vi "main_median_filter_update.vi"(8 "error in (no error)":errorcluster, 9 "Median Filtered Image":T1, 10 "Spaced Out Images":T1[](array[typedef]), 11 "Session In":T2) -> (0 "error out":errorcluster)   [LabVIEW 2019]
uses:
  <vilib>/userDefined/High Color/IMAQdx.ctl
  <vilib>/vision/Image Controls.llb/IMAQ Image.ctl
  <vilib>/vision/driver/IMAQdx.llb/IMAQdx Buffer Number Mode.ctl
  ParametersGlobal.vi
  DebugGlobal.vi
  <vilib>/vision/driver/NI_Vision_Acquisition_Software.lvlib
  <vilib>/vision/NI_Vision_Development_Module.lvlib
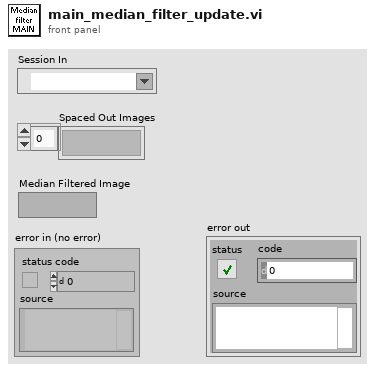
[diagram p1: front panel]
types:
  T1 = typedef "IMAQ Image.ctl" = refnum<image>
  T2 = typedef "IMAQdx.ctl" = refnum<k21>
  T3 = typedef "Image Type" = u32
  T4 = typedef "NI_Vision_Acquisition_Software.lvlib/IMAQdx Buffer Number Mode.ctl" = enum32{"Next", "Last", "Buffer Number", "Every", "Last New"}
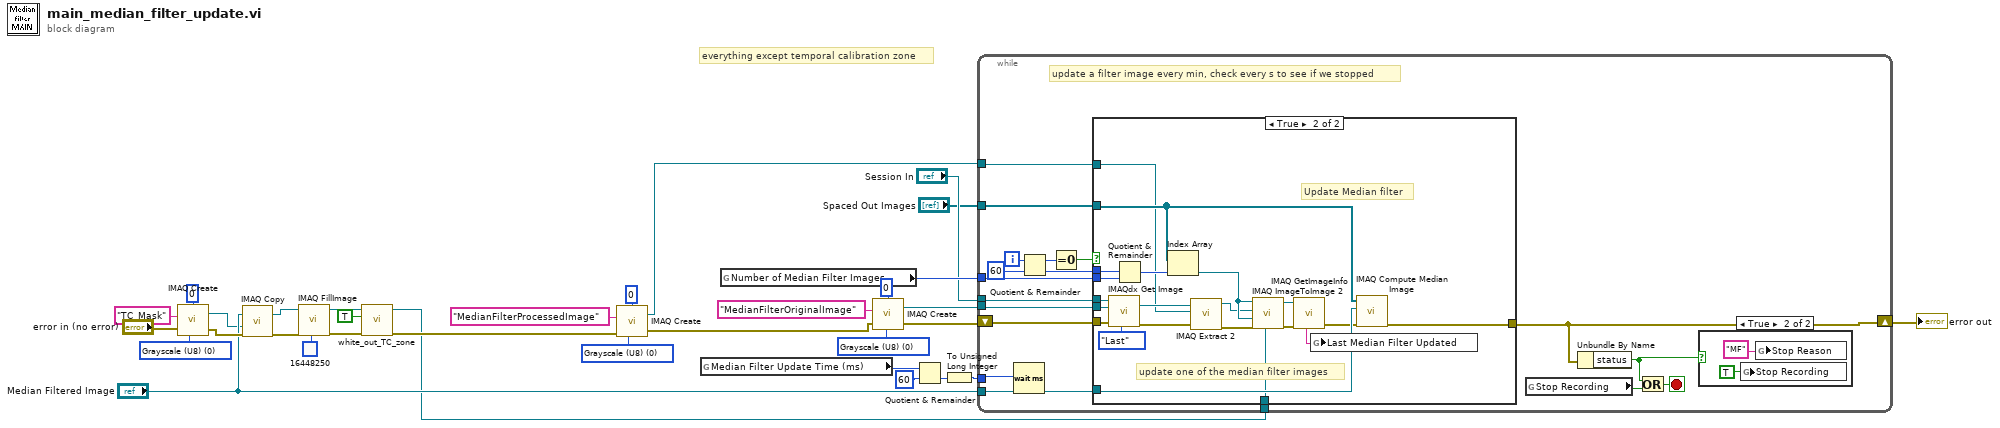
[diagram p0: block diagram]
diagram:
  w13 = T3 0 items=["Grayscale (U8)", "Grayscale (I16)", "Grayscale (SGL)", "Complex (CSG)", "RGB (U32)", "HSL (U32)", "RGB (U64)"] ("Image Type")
  w18 = T3 0 items=["Grayscale (U8)", "Grayscale (I16)", "Grayscale (SGL)", "Complex (CSG)", "RGB (U32)", "HSL (U32)", "RGB (U64)"] ("Image Type")
  w26 = T3 0 items=["Grayscale (U8)", "Grayscale (I16)", "Grayscale (SGL)", "Complex (CSG)", "RGB (U32)", "HSL (U32)", "RGB (U64)"] ("Image Type")
  # "everything except temporal calibration zone"
  n1 = call "IMAQ Create"("Border Size"=0, "Image Name"="TC_Mask", "Image Type"=w13, "error in (no error)"="error in (no error)") -> ("New Image"=w9:T1, "error out"=w11:errorcluster)  [unwired: 1 in]
  n2 = call "IMAQ Copy"("error in (no error)"=w11, "Image Dst"=w9, "Image Src"="Median Filtered Image") -> ("error out"=w7:errorcluster, "Image Dst Out"=w6:T1)  [unwired: 3 in]
  n3 = call "IMAQ FillImage"("Color Pixel Value"=u32 16448250, "error in (no error)"=w7, "Image"=w6) -> ("error out"=w4:errorcluster, "Image Out"=w3:T1)  [unwired: 7 in]
  n4 = call "white_out_TC_zone.vi"("error in (no error)"=w4, "Blackout?"=TRUE, "Refnum in"=w3) -> ("error out"=w2:errorcluster, "Refnum out"=w1:T1)  [unwired: 7 in]
  n5 = call "IMAQ Create"("Border Size"=0, "Image Name"="MedianFilterProcessedImage", "Image Type"=w18, "error in (no error)"=w2) -> ("New Image"=w16:T1, "error out"=w17:errorcluster)  [unwired: 1 in]
  n6 = global read "ParametersGlobal.vi" "Median Filter Update Time (ms)"() -> (w30:i32)
  n7 = global read "ParametersGlobal.vi" "Number of Median Filter Images"() -> (w29:i32)
  n8 = call "IMAQ Create"("Border Size"=0, "Image Name"="MedianFilterOriginalImage", "Image Type"=w26, "error in (no error)"=w17) -> ("New Image"=w27:T1, "error out"=w28:errorcluster)  [unwired: 1 in]
  n9 = Quotient & Remainder(x=w30, y=60 ("milliseconds to wait")) -> (floor(x/y)=w31:i32)  [unwired: 1 out]
  n10 = To Unsigned Long Integer(number=w31) -> (unsigned 32bit integer=w33:u32)
  n11 = while {
    shift-right: [w46] -> w21
    shift-left: w28 -> [w44]
    tunnel: "Session In" -> [w51]
    tunnel: w27 -> [w49]
    tunnel: w29 -> [w48]
    tunnel: w33 -> [w39]
    tunnel: "Median Filtered Image" -> [w45]
    tunnel: "Spaced Out Images" -> [w47]
    tunnel: w16 -> [w35]
    tunnel: w1 -> [w34]
    i -> [w43]
    stop <- w50 stop-if-true
    # "update a filter image every min, check every s to see if we stopped"
    n12 = Wait (ms)(milliseconds to wait=w39) -> ()  [unwired: 1 out]
    n13 = Quotient & Remainder(x=w43, y=60 ("milliseconds to wait")) -> (x-y*floor(x/y)=w40:i32, floor(x/y)=w41:i32)
    n14 = Equal To 0?(x=w40) -> (x = 0?=w42:bool)
    n15 = case shown="True" w42 {
      tunnel: w51 -> [_ w74]
      tunnel: w49 -> [_ w73]
      tunnel: w41 -> [_ w72]
      tunnel: w48 -> [_ w71]
      tunnel: w47 -> [_ w64]
      tunnel: [w54 w56] -> w46
      tunnel: w45 -> [_ w69]
      tunnel: w44 -> [w54 w68]
      tunnel: w35 -> [_ w57]
      tunnel: w34 -> [_ w55]
      frame False {
      }
      frame True {
        # "Update Median filter"
        # "update one of the median filter images"
        n16 = call <vilib>:"IMAQdx Get Image.vi"("Buffer Number Mode (Next)"=IMAQdx_Buffer_Number_Mode."Last", "error in"=w68, "Image In"=w73, "Session In"=w74) -> ("error out"=w62:errorcluster, "Image Out"=w58:T1)  [unwired: 4 in, 2 out]
        n17 = Quotient & Remainder(x=w72, y=w71) -> (x-y*floor(x/y)=w70:i32)  [unwired: 1 out]
        n18 = Index Array(array=w64, index=w70) -> (element=w66:T1)
        n19 = call "IMAQ Extract 2"("error in (no error)"=w62, "Image Dst"=w57, "Image Src"=w58) -> ("error out"=w67:errorcluster, "Image Dst Out"=w65:T1)  [unwired: 7 in]
        n20 = call "IMAQ ImageToImage 2"("Image Mask"=w55, "error in (no error)"=w67, "Image Dst"=w66, "Image Src (Small)"=w65, "Image Src (Large)"=w66) -> ("error out"=w61:errorcluster, "Image Dst Out"=w59:T1)  [unwired: 5 in]
        n21 = call "IMAQ GetImageInfo"("error in (no error)"=w61, "Image"=w59) -> ("error out"=w60:errorcluster, "Image Name"=w63:string)  [unwired: 2 in, 6 out]
        n22 = global write "DebugGlobal.vi" "Last Median Filter Updated"(w63) -> ()
        n23 = call "IMAQ Compute Median Image"("error in (no error)"=w60, "Image Dst"=w69, "Images"=w64) -> ("error out"=w56:errorcluster)  [unwired: 7 in, 1 out]
      }
    }
    n24 = global read "DebugGlobal.vi" "Stop Recording"() -> (w36:bool)
    n25 = Unbundle By Name(w46) -> ("status"=w37:bool)
    n26 = Or(x=w37, y=w36) -> (x .or. y?=w50:bool)
    n27 = case shown="True" w37 {
      frame False {
      }
      frame True {
        n28 = global write "DebugGlobal.vi" "Stop Recording"(TRUE ("stop")) -> ()
        n29 = global write "DebugGlobal.vi" "Stop Reason"("MF" ("Stop Debug")) -> ()
      }
    }
  }
  "error out" <- w21
